vi "Get Color.vi"(11 "Point":refnum<class "Point.lvclass">) -> (3 "Color":u32(colorbox))   [LabVIEW 2018, in "Point.lvclass"]
doc: "Get the point's color."
uses:
  Point.lvclass
  Point.lvclass/Point.ctl
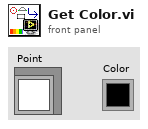
[diagram p1: front panel]
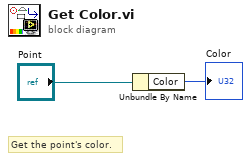
[diagram p0: block diagram]
diagram:
  # "Get the point's color."
  n1 = Unbundle By Name("Point") -> ("Color"=→"Color":u32)
